vi "Serial_Read_with_Timeout_re.vi"(3 "Bytes to Read":u32=10 caption="“Ç‚ÝŽæ‚èÊÞ²Ä", 4 "Timeout Limit":dbl=5.0 caption="À²Ñ±³Ä§À" format="%.2f", 5 "Port Number":i32=1 caption="Îß°ÄÔ") -> (0 "Error Out":bool caption="´×°", 1 "Timeout":bool caption="啦驯衬", 2 "Serial Read":string caption="¼Ø±Ù“Ç‚ÝŽæ‚è")   [LabVIEW 2016]
doc: "±ÌVIÅÍóM·éÃÞ°ÀÌÊÞ²ÄÆÃÞ°ÀðÒ@·é§ÀÔðÝèµÜ·B§ÀÔàÉwè³ê½ÊÞ²ÄÌÃÞ°ÀðóMµÈ©Á½êAÃÞ°ÀðßµÜ¹ñBOÃÞ°ÀðóMµ½êÍ¦É·×ÄÌÃÞ°ÀðßµÜ·B"
panel:
  # "PC:  0 = COM1, 1= COM2,...\nMac:  0 = Modem, 1 = Printer\nSun: 0 = ttya, 1 = ttyb,..."
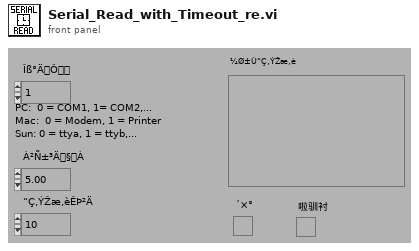
[diagram p1: front panel]
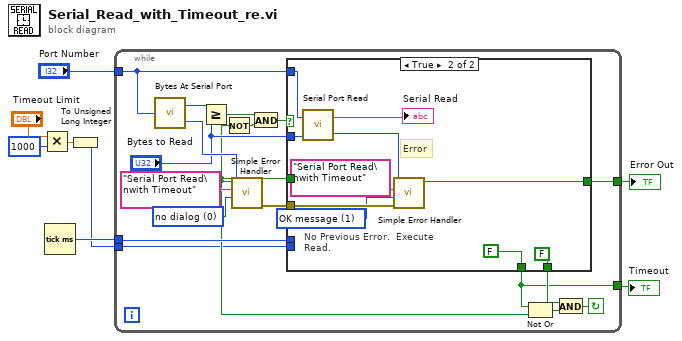
[diagram p0: block diagram]
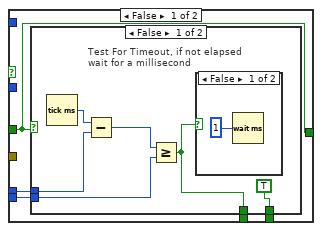
[diagram p2: hidden frame]
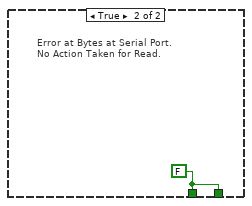
[diagram p4: hidden frame]
diagram:
  n1 = Multiply(x="Timeout Limit", y=u32 1000) -> (x*y=w2:dbl)
  n2 = Tick Count (ms)() -> (millisecond timer value=w7:u32)
  n3 = To Unsigned Long Integer(number=w2) -> (unsigned 32bit integer=w1:u32)
  n4 = while {
    tunnel: w1 -> [w9]
    tunnel: [w11] -> w5
    tunnel: [w23] -> w6
    tunnel: w7 -> [w12]
    tunnel: "Port Number" -> [w19]
    stop <- w13 continue-if-true
    w17 = 0 items=["no dialog", "OK message", "continue or stop message"] ("type of dialog (OK msg:1)")
    n5 = call <vilib>:"Bytes At Serial Port.vi"("port number"=w19) -> ("byte count"=w26:u32, "error code"=w25:i32)
    n6 = Greater Or Equal?(x=w26, y="Bytes to Read") -> (x >= y?=w21:bool)
    n7 = call <vilib>:"Simple Error Handler.vi"("error code (no error:0)"=w25, "error source (\" \")"="Serial Port Read\nwith Timeout", "type of dialog (OK msg:1)"=w17) -> ("error?"=w10:bool, "error out"=w18:errorcluster)  [unwired: 1 in, 4 out]
    n8 = Not(x=w10) -> (.not. x?=w20:bool)
    n9 = And(x=w21, y=w20) -> (x .and. y?=w22:bool)
    n10 = case shown="True" w22 {
      tunnel: w19 -> [_ w45]
      tunnel: "Bytes to Read" -> [_ w49]
      tunnel: [w29 w46] -> w23
      tunnel: w10 -> [w29 _]
      tunnel: w18 -> [_ w44]
      tunnel: [w31 FALSE] -> w14
      tunnel: w12 -> [w30 _]
      tunnel: [w28 FALSE] -> w11
      tunnel: w9 -> [w27 _]
      frame False {
        n11 = case shown="False" w29 {
          tunnel: [TRUE w39] -> w31
          tunnel: w30 -> [w35 _]
          tunnel: [w34 w39] -> w28
          tunnel: w27 -> [w32 _]
          frame False {
            # "Test For Timeout, if not elapsed\nwait for a millisecond"
            n12 = Tick Count (ms)() -> (millisecond timer value=w36:u32)
            n13 = Subtract(x=w36, y=w35) -> (x-y=w33:u32)
            n14 = Greater Or Equal?(x=w33, y=w32) -> (x >= y?=w34:bool)
            n15 = case shown="False" w34 {
              frame False {
                n16 = Wait (ms)(milliseconds to wait=u32 1 ("f")) -> ()  [unwired: 1 out]
              }
              frame True {
              }
            }
          }
          frame True {
            w39 = FALSE
            # "Error at Bytes at Serial Port.\nNo Action Taken for Read."
          }
        }
      }
      frame True {
        w40 = 1 items=["no dialog", "OK message", "continue or stop message"] ("type of dialog (OK msg:1)")
        # "No Previous Error.  Execute\nRead."
        # "Error"
        n17 = call <vilib>:"Serial Port Read.vi"("requested byte count"=w49, "port number"=w45) -> ("error code"=w47:i32, "string read"=→"Serial Read":string)
        n18 = call <vilib>:"Simple Error Handler.vi"("error code (no error:0)"=w47, "error source (\" \")"="Serial Port Read\nwith Timeout", "type of dialog (OK msg:1)"=w40, "error in (no error)"=w44) -> ("error?"=w46:bool)  [unwired: 5 out]
      }
    }
    n19 = Not Or(1:w10, 2:w11) -> (0:w15:bool)
    n20 = And(x=w14, y=w15) -> (x .and. y?=w13:bool)
  }
  "Error Out" <- w6
  "Timeout" <- w5
